vi "test-cubic-spline-03.vi"() -> (3 "Test Passed":bool)   [LabVIEW 2019]
uses:
  <vilib>/Rock Robotics/WPI/ThirdParty/JAS_Junk/TrajLib/POSEwCURVATURE.ctl
  <vilib>/Rock Robotics/WPI/ThirdParty/JAS_Junk/TrajLib/POSE2D.ctl
  <vilib>/Rock Robotics/WPI/ThirdParty/JAS_Junk/TrajLib/TRANSLATION2D.ctl
  <vilib>/Rock Robotics/WPI/ThirdParty/JAS_Junk/TrajLib/ROTATION2D.ctl
  <vilib>/Rock Robotics/WPI/ThirdParty/JAS_Junk/TrajLib/Rotation_CreateAngle.vi
  <vilib>/Rock Robotics/WPI/ThirdParty/JAS_Junk/TrajLib/Util_CalcDist.vi
  <vilib>/Rock Robotics/WPI/ThirdParty/JAS_Junk/TrajLib/Trajectory_Library.lvlib
panel:
  out "XY Graph":cluster{dbl[], dbl[]}(graph)
  out "All Interior \nwayPoints\nFound (True)":bool
  out "end rot = 0":dbl
  out "end y = 0":dbl
  out "end x = 0":dbl
  out "start rot = 0":dbl
  out "start y = 0":dbl
  out "start x = 0":dbl
  out "max dtheta < 0.0872":dbl
  out "max dy < 0.00127":dbl
  out "max dx  < 0.127":dbl
  out "Overall Error":errorcluster
  out "Elements":i32
  out "Create Spline Error":errorcluster
  out "SplinePoses\nWCurve":T1[](array[typedef]) {"POSE"."ROTATION"."SIN" format="%13.4f"; "POSE"."ROTATION"."COS" format="%13.4f"; "POSE"."ROTATION"."VALUE" format="%13.4f"; "POSE"."TRANSLATION"."Y" format="%14.3f"; "POSE"."TRANSLATION"."X" format="%14.3f"}
  out "Elapsed Time":dbl
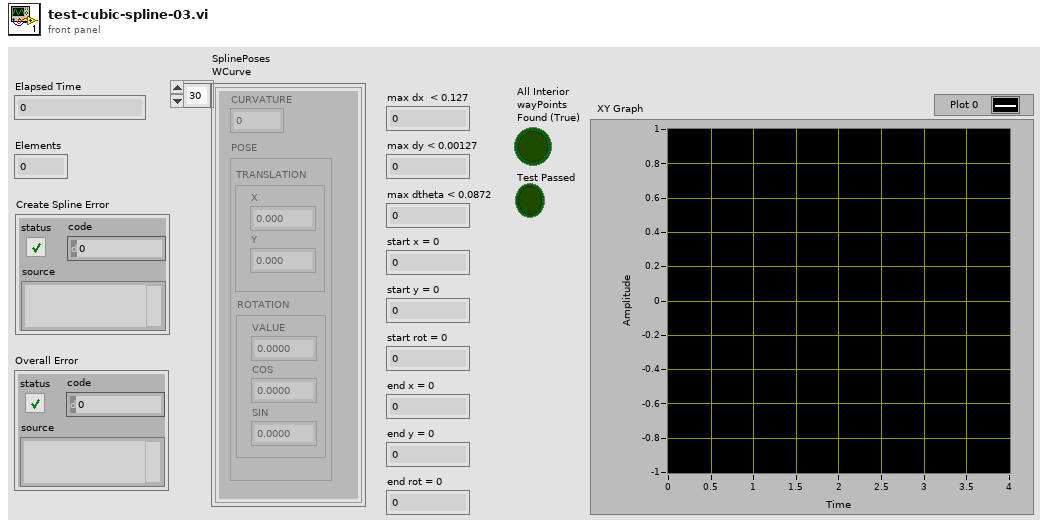
[diagram p1: front panel]
types:
  T1 = typedef "Trajectory_Library.lvlib/POSEwCURVATURE.ctl" = cluster{"CURVATURE":dbl, "POSE":T2}
  T2 = typedef "Trajectory_Library.lvlib/POSE2D.ctl" = cluster{"TRANSLATION":T3, "ROTATION":T4}
  T3 = typedef "Trajectory_Library.lvlib/TRANSLATION2D.ctl" = cluster{"X":dbl, "Y":dbl}
  T4 = typedef "Trajectory_Library.lvlib/ROTATION2D.ctl" = cluster{"VALUE":dbl, "COS":dbl, "SIN":dbl}
  T5 = typedef "Trajectory_Library.lvlib/SPLINE_CTRL_VECTOR.ctl" = cluster{"Xs":dbl[], "Ys":dbl[]}
  T6 = typedef "Trajectory_Library.lvlib/SPLINE.ctl" = cluster{"Degree":i32, "Coefficients":T7}
  T7 = typedef "NI_Matrix.lvlib/RealMatrix.ctl" = dbl[][]
  T8 = typedef "Trajectory_Library.lvlib/TWIST2D.ctl" = cluster{"dX":dbl, "dY":dbl, "dTHETA":dbl}
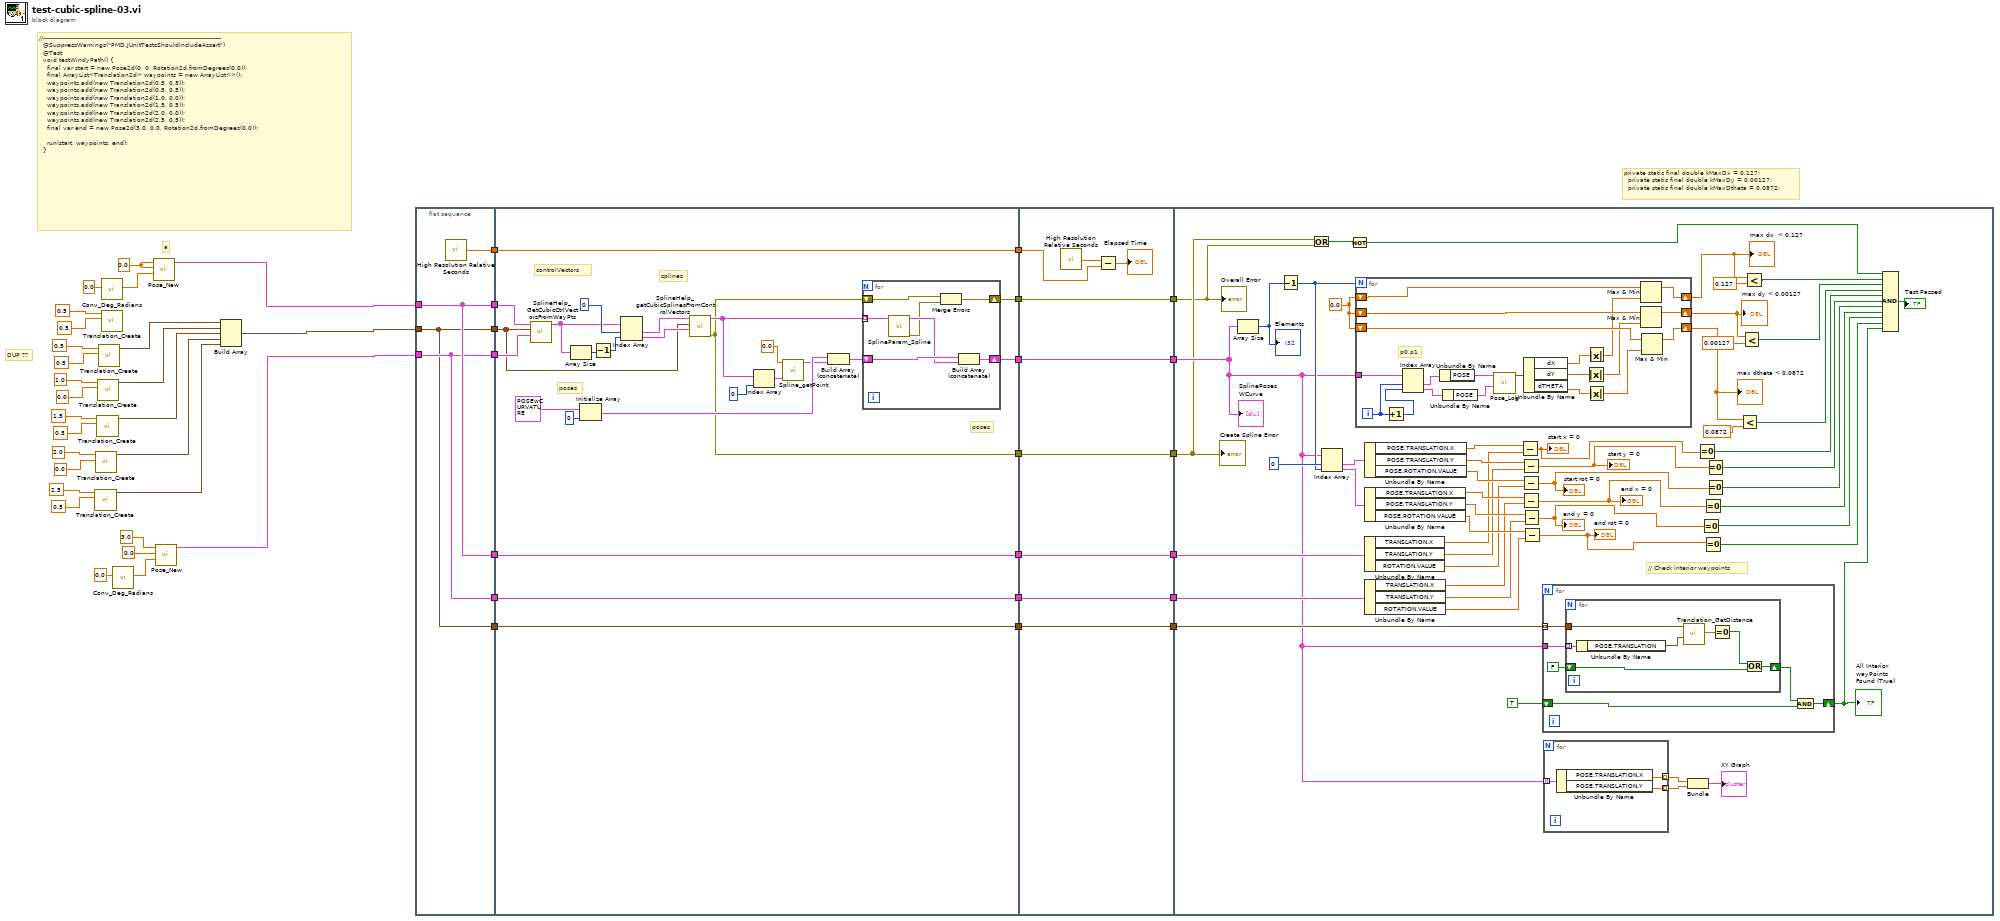
[diagram p0: block diagram]
diagram:
  w25 = 0.0 ("X")
  # "DUP ??"
  # "a"
  # "//-----------------------------------------------------------------------------------------\n  @SuppressWarnings(\"PMD.JUnitTestsShouldIncludeAssert\")\n  @Test\n  void testWindyPath() {\n    final var start = new Pose2d(0, 0, Rotation2d.fromDegrees(0.0));\n    final ArrayList<Translation2d> waypoints = new ArrayList<>();\n    waypoints.add(new Translation2d(0.5, 0.5));\n    waypoints.add(new Translation2d(0.5, 0.5));\n    waypoints.add(new Translation2d(1.0, 0.0));\n    waypoints.add(new Translation2d(1.5, 0.5));\n    waypoints.add(new Translation2d(2.0, 0.0));\n    waypoints.add(new Translation2d(2.5, 0.5));\n    final var end = new Pose2d(3.0, 0.0, Rotation2d.fromDegrees(0.0));\n\n    run(start, waypoints, end);\n  }"
  # "private static final double kMaxDx = 0.127;\n  private static final double kMaxDy = 0.00127;\n  private static final double kMaxDtheta = 0.0872;"
  n1 = call <vilib>:"Translation_Create.vi"("Y"=0.5, "X"=2.5) -> ("TRANSLATION"=w4:T3)  [unwired: 9 in]
  n2 = call <vilib>:"Translation_Create.vi"("Y"=0.0, "X"=2.0) -> ("TRANSLATION"=w5:T3)  [unwired: 9 in]
  n3 = call <vilib>:"Translation_Create.vi"("Y"=0.5, "X"=1.5) -> ("TRANSLATION"=w6:T3)  [unwired: 9 in]
  n4 = call <vilib>:"Translation_Create.vi"("Y"=0.0, "X"=1.0) -> ("TRANSLATION"=w7:T3)  [unwired: 9 in]
  n5 = call <vilib>:"Translation_Create.vi"("Y"=0.5, "X"=0.5) -> ("TRANSLATION"=w8:T3)  [unwired: 9 in]
  n6 = call <vilib>:"Conv_Deg_Radians.vi"("Degress"=0.0) -> ("Radians"=w24:dbl)  [unwired: 10 in]
  n7 = call <vilib>:"Translation_Create.vi"("Y"=0.5, "X"=0.5) -> ()  [unwired: 9 in, 1 out]
  n8 = call <vilib>:"Conv_Deg_Radians.vi"("Degress"=0.0) -> ("Radians"=w19:dbl)  [unwired: 10 in]
  n9 = call <vilib>:"Pose_New.vi"("Heading"=w24, "Y"=w25, "X"=w25) -> ("out POSe"=w3:T2)  [unwired: 8 in]
  n10 = call <vilib>:"Pose_New.vi"("Heading"=w19, "Y"=0.0, "X"=3.0) -> ("out POSe"=w1:T2)  [unwired: 8 in]
  n11 = Build Array(w8, w7, w6, w5, w4) -> (w2:T3[])
  n12 = flat-sequence {
    tunnel: w3 -> [w50]
    tunnel: [w50] -> w47
    tunnel: w2 -> [w48]
    tunnel: [w48] -> w46
    tunnel: w1 -> [w49]
    tunnel: [w49] -> w45
    tunnel: [w51] -> w44
    tunnel: [w50] -> w36
    tunnel: [w49] -> w33
    tunnel: [w48] -> w28
    tunnel: w47 -> [w76]
    tunnel: w46 -> [w68]
    tunnel: w45 -> [w75]
    tunnel: [w67] -> w43
    tunnel: w44 -> [w67]
    tunnel: [w57] -> w42
    tunnel: [w56] -> w40
    tunnel: [w55] -> w38
    tunnel: w36 -> [w54]
    tunnel: [w54] -> w35
    tunnel: w33 -> [w53]
    tunnel: [w53] -> w32
    tunnel: [w52] -> w29
    tunnel: w28 -> [w52]
    tunnel: w43 -> [w92]
    tunnel: w42 -> [w91]
    tunnel: [w91] -> w41
    tunnel: w40 -> [w90]
    tunnel: [w90] -> w39
    tunnel: w38 -> [w89]
    tunnel: [w89] -> w37
    tunnel: w35 -> [w86]
    tunnel: [w86] -> w34
    tunnel: w32 -> [w85]
    tunnel: [w85] -> w31
    tunnel: [w84] -> w30
    tunnel: w29 -> [w84]
    tunnel: w41 -> [w120]
    tunnel: w39 -> [w95]
    tunnel: w37 -> [w94]
    tunnel: w34 -> [w143]
    tunnel: w31 -> [w142]
    tunnel: w30 -> [w125]
    frame #0 {
      n13 = call <vilib>:"High Resolution Relative Seconds.vi"() -> ("relative seconds"=w51:dbl)
    }
    frame #1 {
      # "poses"
      # "poses"
      # "splines"
      # "controlVectors"
      n14 = call <vilib>:"SplineHelp_GetCubicCtrlVectorsFromWayPts.vi"("Enging POSE"=w75, "Interior WAYPOINTS"=w68, "Starting POSE"=w76) -> ("SplineControlVectors"=w72:T5[])  [unwired: 8 in]
      n15 = Array Size(array=w72) -> (size(s)=w73:i32)
      n16 = Initialize Array(T1 {"CURVATURE"=0.0, "POSE"={"TRANSLATION"={"X"=0.0, "Y"=0.0}, "ROTATION"={"VALUE"=0.0, "COS"=1.0, "SIN"=0.0}}} ("POSEwCURVATURE"), 0 ("dimension size")) -> (w61:T1[])
      n17 = Decrement(x=w73) -> (x-1=w71:i32)
      n18 = Index Array(array=w72, index #1=0 ("index"), index #2=w71) -> (element #1=w70:T5, element #2=w69:T5)
      n19 = call <vilib>:"SplineHelp_getCubicSplinesFromControlVectors.vi"("endCtrlVector"=w69, "InternalWaypoints"=w68, "startCtrlVector"=w70) -> ("error out"=w56:errorcluster, "splines"=w58:T6[])  [unwired: 3 in, 4 out]
      n20 = Index Array(array=w58, index=0) -> (element=w63:T6)
      n21 = call <vilib>:"Spline_getPoint.vi"("inputSPLINE"=w63, "Time"=0.0) -> ("POSEwCURVATURE"=w60:T1)  [unwired: 9 in]
      n22 = Build Array (concatenate)(w61, w60) -> (w59:T1[])
      n23 = for {
        shift-right: [w80] -> w57
        shift-left: w59 -> [w82]
        tunnel: w58 -> [w83] mode=indexing
        shift-right: [w78] -> w55
        shift-left: w56 -> [w79]
        n24 = call <vilib>:"SplineParam_Spline.vi"("inputSPLINE"=w83) -> ("error out"=w77:errorcluster, "outputPOSEwCURVATURE"=w81:T1[])  [unwired: 9 in]
        n25 = Merge Errors(w79, w77) -> (w78:errorcluster)
        n26 = Build Array (concatenate)(w82, w81) -> (w80:T1[])
      }
    }
    frame #2 {
      n27 = call <vilib>:"High Resolution Relative Seconds.vi"() -> ("relative seconds"=w87:dbl)
      n28 = Subtract(x=w87, y=w92) -> (x-y=→"Elapsed Time":dbl)
    }
    frame #3 {
      w144 = 0.0
      # "// Check interior waypoints"
      n29 = Array Size(array=w120) -> (size(s)=w145:i32)
      "Elements" <- w145
      n30 = Decrement(x=w145) -> (x-1=w140:i32)
      n31 = Or(x=w95, y=w94) -> (x .or. y?=w96:bool)
      n32 = Index Array(array=w120, index #1=0 ("index"), index #2=w140) -> (element #1=w139:T1, element #2=w138:T1)
      n33 = Not(x=w96) -> (.not. x?=w93:bool)
      n34 = for {
        N: w140 -> [_]
        tunnel: w120 -> [w179]
        shift-right: [w170] -> w117
        shift-left: w144 -> [w167]
        shift-right: [w168] -> w119
        shift-left: w144 -> [w165]
        shift-right: [w169] -> w118
        shift-left: w144 -> [w166]
        i -> [w181]
        # "p0,p1"
        n35 = Increment(x=w181) -> (x+1=w180:i32)
        n36 = Index Array(array=w179, index #1=w181, index #2=w180) -> (element #1=w178:T1, element #2=w177:T1)
        n37 = Unbundle By Name(w178) -> ("POSE"=w176:T2)
        n38 = Unbundle By Name(w177) -> ("POSE"=w175:T2)
        n39 = call <vilib>:"Pose_Log.vi"("end POSE"=w175, "in POSE"=w176) -> ("out TWIST"=w174:T8)  [unwired: 9 in]
        n40 = Unbundle By Name(w174) -> ("dX"=w171:dbl, "dY"=w172:dbl, "dTHETA"=w173:dbl)
        n41 = Absolute Value(x=w172) -> (abs(x)=w163:dbl)
        n42 = Absolute Value(x=w171) -> (abs(x)=w164:dbl)
        n43 = Absolute Value(x=w173) -> (abs(x)=w162:dbl)
        n44 = Max & Min(x=w167, y=w164) -> (max(x,y)=w170:dbl)  [unwired: 1 out]
        n45 = Max & Min(x=w166, y=w163) -> (max(x,y)=w169:dbl)  [unwired: 1 out]
        n46 = Max & Min(x=w165, y=w162) -> (max(x,y)=w168:dbl)  [unwired: 1 out]
      }
      "max dx  < 0.127" <- w117
      "max dy < 0.00127" <- w118
      "max dtheta < 0.0872" <- w119
      n47 = Unbundle By Name(w138) -> ("POSE.TRANSLATION.X"=w134:dbl, "POSE.TRANSLATION.Y"=w133:dbl, "POSE.ROTATION.VALUE"=w132:dbl)
      n48 = Unbundle By Name(w143) -> ("TRANSLATION.X"=w131:dbl, "TRANSLATION.Y"=w130:dbl, "ROTATION.VALUE"=w129:dbl)
      n49 = Unbundle By Name(w139) -> ("POSE.TRANSLATION.X"=w137:dbl, "POSE.TRANSLATION.Y"=w136:dbl, "POSE.ROTATION.VALUE"=w135:dbl)
      n50 = Unbundle By Name(w142) -> ("TRANSLATION.X"=w128:dbl, "TRANSLATION.Y"=w127:dbl, "ROTATION.VALUE"=w126:dbl)
      n51 = Subtract(x=w137, y=w131) -> (x-y=w110:dbl)
      "start x = 0" <- w110
      n52 = Subtract(x=w136, y=w130) -> (x-y=w109:dbl)
      "start y = 0" <- w109
      n53 = Subtract(x=w135, y=w129) -> (x-y=w108:dbl)
      "start rot = 0" <- w108
      n54 = Subtract(x=w134, y=w128) -> (x-y=w107:dbl)
      "end x = 0" <- w107
      n55 = Subtract(x=w133, y=w127) -> (x-y=w106:dbl)
      "end y = 0" <- w106
      n56 = Subtract(x=w132, y=w126) -> (x-y=w105:dbl)
      "end rot = 0" <- w105
      n57 = for {
        tunnel: w125 -> [w149] mode=indexing
        tunnel: w120 -> [w154]
        shift-right: [w153] -> w98
        shift-left: TRUE -> [w152]
        n58 = for {
          tunnel: w154 -> [w158] mode=indexing
          shift-right: [w161] -> w150
          shift-left: FALSE -> [w160]
          tunnel: w149 -> [w159]
          n59 = Unbundle By Name(w158) -> ("POSE.TRANSLATION"=w157:T3)
          n60 = call <vilib>:"Translation_GetDistance.vi"("other Translation"=w157, "In Translation"=w159) -> ("Distance"=w156:dbl)  [unwired: 9 in]
          n61 = Equal To 0?(x=w156) -> (x = 0?=w155:bool)
          n62 = Or(x=w155, y=w160) -> (x .or. y?=w161:bool)
        }
        n63 = And(x=w150, y=w152) -> (x .and. y?=w153:bool)
      }
      "All Interior \nwayPoints\nFound (True)" <- w98
      n64 = for {
        tunnel: [w148] -> w123 mode=indexing
        tunnel: [w147] -> w122 mode=indexing
        tunnel: w120 -> [w146] mode=indexing
        n65 = Unbundle By Name(w146) -> ("POSE.TRANSLATION.X"=w148:dbl, "POSE.TRANSLATION.Y"=w147:dbl)
      }
      n66 = Bundle(w123, w122) -> (→"XY Graph":cluster{dbl[], dbl[]})  [unwired: 1 in]
      n67 = Equal To 0?(x=w110) -> (x = 0?=w104:bool)
      n68 = Equal To 0?(x=w106) -> (x = 0?=w100:bool)
      n69 = Equal To 0?(x=w107) -> (x = 0?=w101:bool)
      n70 = Equal To 0?(x=w105) -> (x = 0?=w99:bool)
      n71 = Equal To 0?(x=w109) -> (x = 0?=w103:bool)
      n72 = Equal To 0?(x=w108) -> (x = 0?=w102:bool)
      n73 = Less?(x=w119, y=0.0872) -> (x < y?=w111:bool)
      n74 = Less?(x=w118, y=0.00127) -> (x < y?=w112:bool)
      n75 = Less?(x=w117, y=0.127) -> (x < y?=w113:bool)
      n76 = Compound Arithmetic op=AND(w93, w113, w112, w111, w104, w103, w102, w101, w100, w99, w98) -> (→"Test Passed":bool)
      "SplinePoses\nWCurve" <- w120
      "Create Spline Error" <- w95
      "Overall Error" <- w94
    }
  }
